vi "HardWareLoop.vi"(8 "error in (no error)":errorcluster, 10 "ctrls":T2, 11 "Queue cluster":T1) -> ()   [LabVIEW 2017]
uses:
  controls_main.ctl
  QueueCluster.ctl
  EventQueueCluster.ctl
  EventMessage.ctl
  MeasureQueue.ctl
  MeasureMessage.ctl
  HardwareQueueCluster.ctl
  hardwareMessage.ctl
  GUIQueueCluster.ctl
  GUIMessage.ctl
  SaveQueueCluster.ctl
  SaveMessage.ctl
  <vilib>/LabVIEW Interface for Arduino/Type Defs/Arduino Resource.ctl
  <vilib>/LabVIEW Interface for Arduino/Type Defs/Board Type.ctl
  <vilib>/LabVIEW Interface for Arduino/LabVIEW Interface for Arduino.lvlib
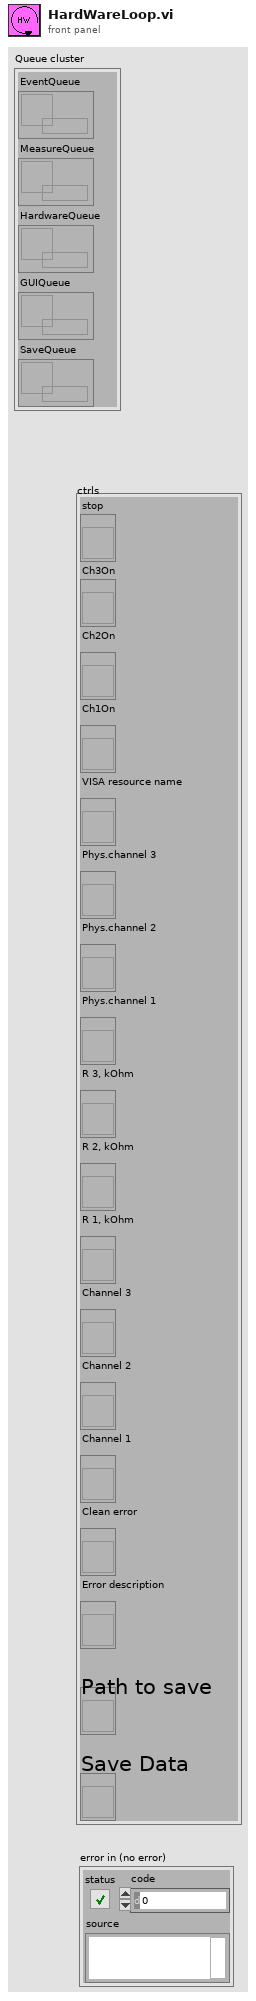
[diagram p1: front panel]
types:
  T1 = typedef "QueueCluster.ctl" = cluster{"EventQueue":refnum<queue>, "MeasureQueue":refnum<queue>, "HardwareQueue":refnum<queue>, "GUIQueue":refnum<queue>, "SaveQueue":refnum<queue>}
  T2 = typedef "controls_main.ctl" = cluster{"stop":refnum<vi>, "Ch3On":refnum<vi>, "Ch2On":refnum<vi>, "Ch1On":refnum<vi>, "VISA resource name":refnum<vi>, "Phys.channel 3":refnum<vi>, "Phys.channel 2":refnum<vi>, "Phys.channel 1":refnum<vi>, "R 3, kOhm":refnum<vi>, "R 2, kOhm":refnum<vi>, "R 1, kOhm":refnum<vi>, "Channel 3":refnum<vi>, "Channel 2":refnum<vi>, "Channel 1":refnum<vi>, "Clean error":refnum<vi>, "Error description":refnum<vi>, "Path to save":refnum<vi>, "Save Data":refnum<vi>}
  T3 = typedef "LabVIEW Interface for Arduino.lvlib/Arduino Resource.ctl" = cluster{"VISA resource":refnum<visa-resource-name>, "Board Type":T4, "Connection Type":enum8{"USB / Serial"}, "Bytes Per Packet (15)":u8}
  T4 = typedef "LabVIEW Interface for Arduino.lvlib/Board Type.ctl" = enum16{"Uno", "Dimuelanove w/Atmega 328", "Mega 2560"}
  T5 = typedef "GUIMessage.ctl" = enum16{"StopSave", "Channel1Value", "Channel2Value", "Channel3Value", "ErrorSource", "CleanError", "StartChannel1", "StartChannel2", "StartChannel3", "StopChannel1", "StopChannel2", "StopChannel3", "Halt"}
  T6 = typedef "GUIQueueCluster.ctl" = cluster{"GUIMessage":T5, "NumericValue":dbl, "String":string}
  T7 = typedef "HardwareQueueCluster.ctl" = cluster{"HardwareMessage":T8, "NumericValue":dbl, "String":string}
  T8 = typedef "hardwareMessage.ctl" = enum16{"Init", "MeasureChannel", "CloseDevice", "Error", "Halt", "SetPhysChannel1", "SetPhysChannel2", "SetPhysChannel3"}
  T9 = typedef "SaveMessage.ctl" = enum16{"StartSaving", "StopSaving", "Ch1Value", "Ch2Value", "Ch3Value", "Error", "WriteFile", "Halt"}
  T10 = typedef "SaveQueueCluster.ctl" = cluster{"Save message":T9, "NumericValue":dbl, "String":string}
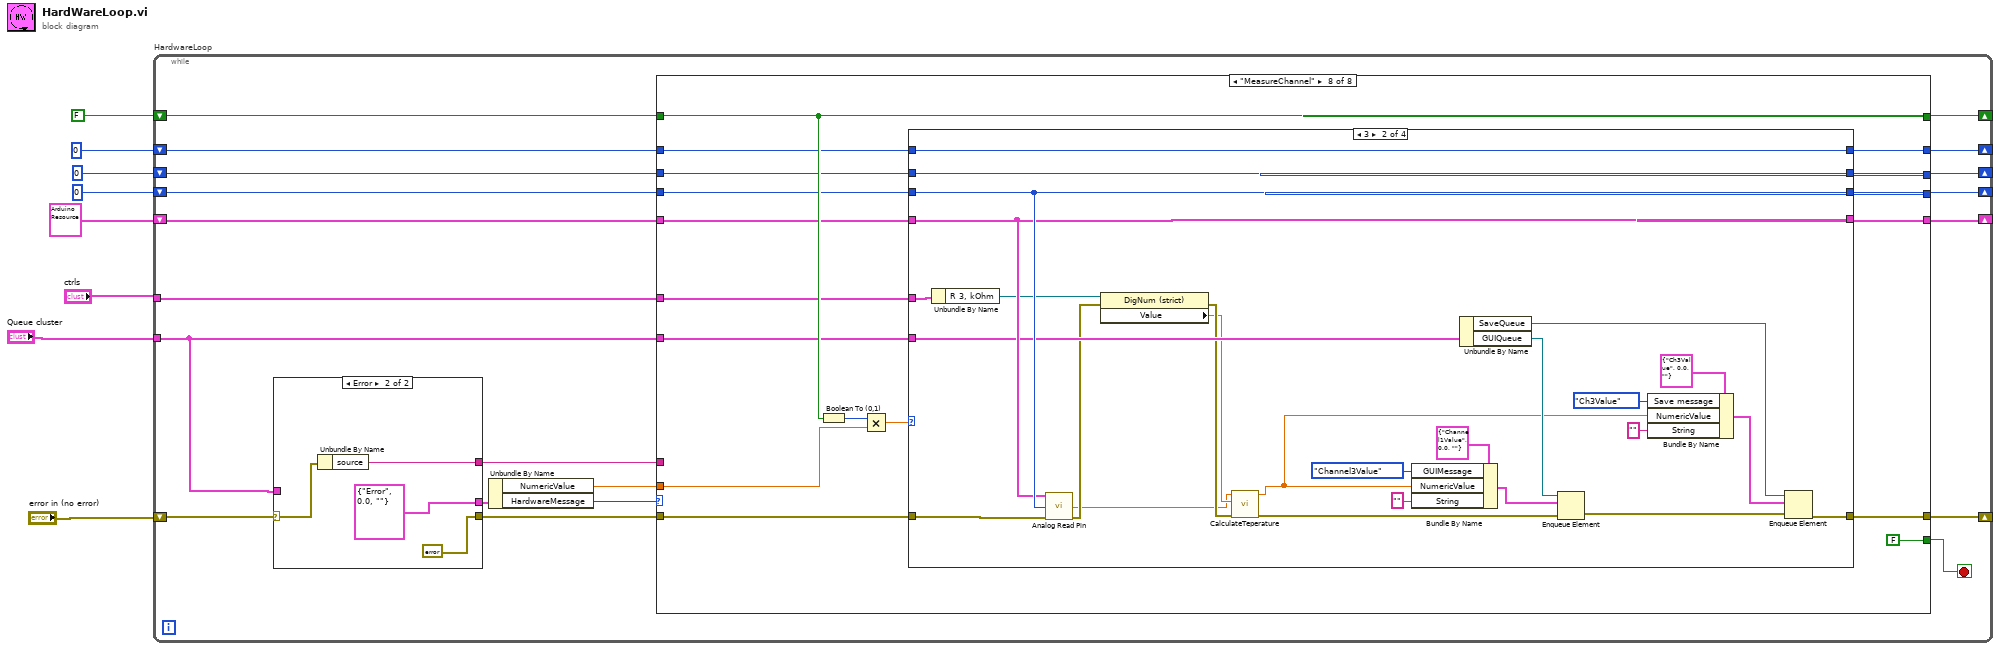
[diagram p0: block diagram]
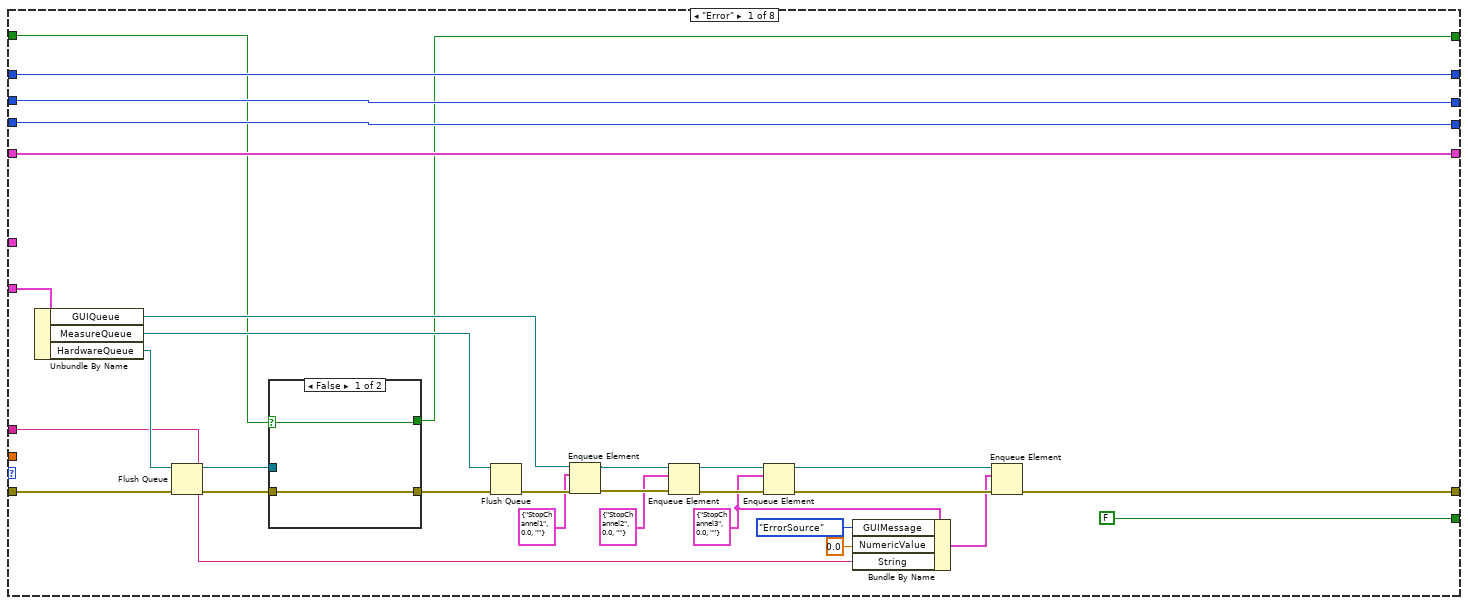
[diagram p2: hidden frame]
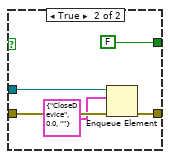
[diagram p3: hidden frame]
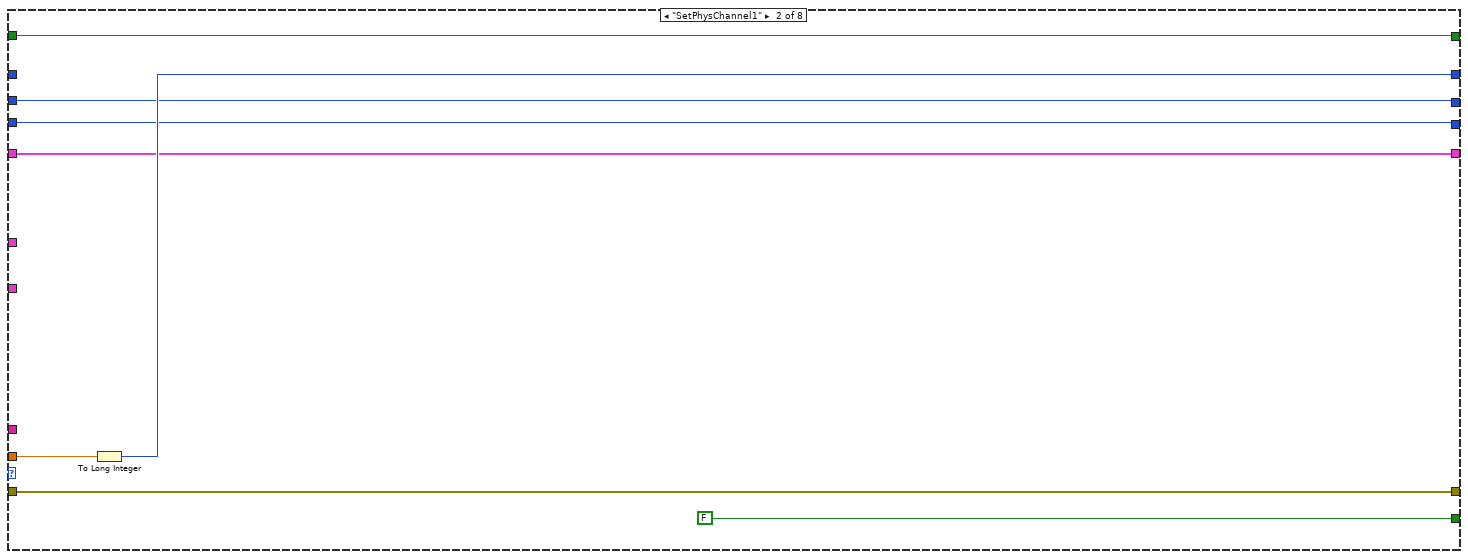
[diagram p4: hidden frame]
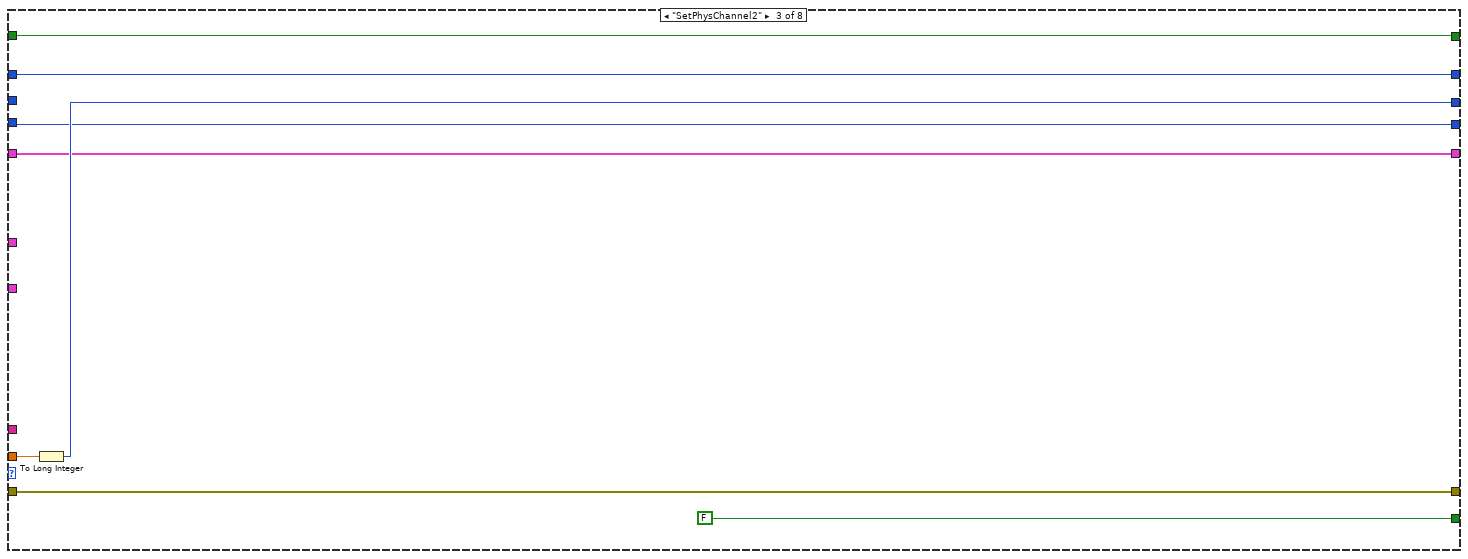
[diagram p5: hidden frame]
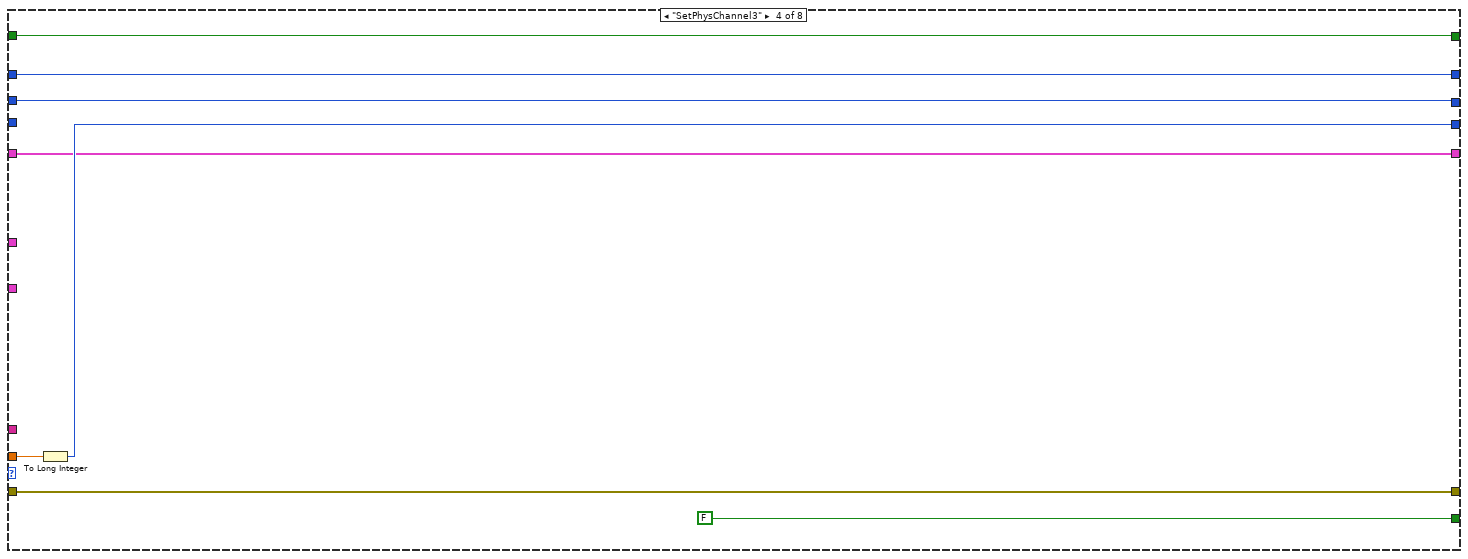
[diagram p6: hidden frame]
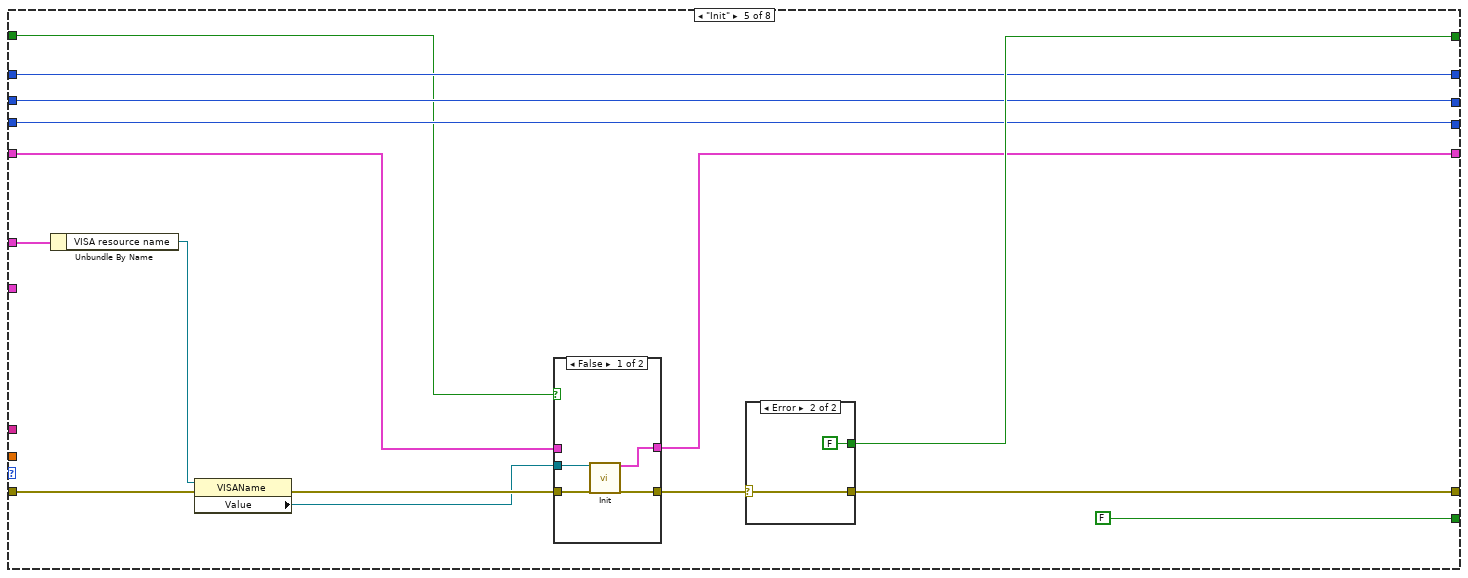
[diagram p7: hidden frame]
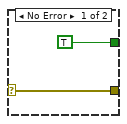
[diagram p9: hidden frame]
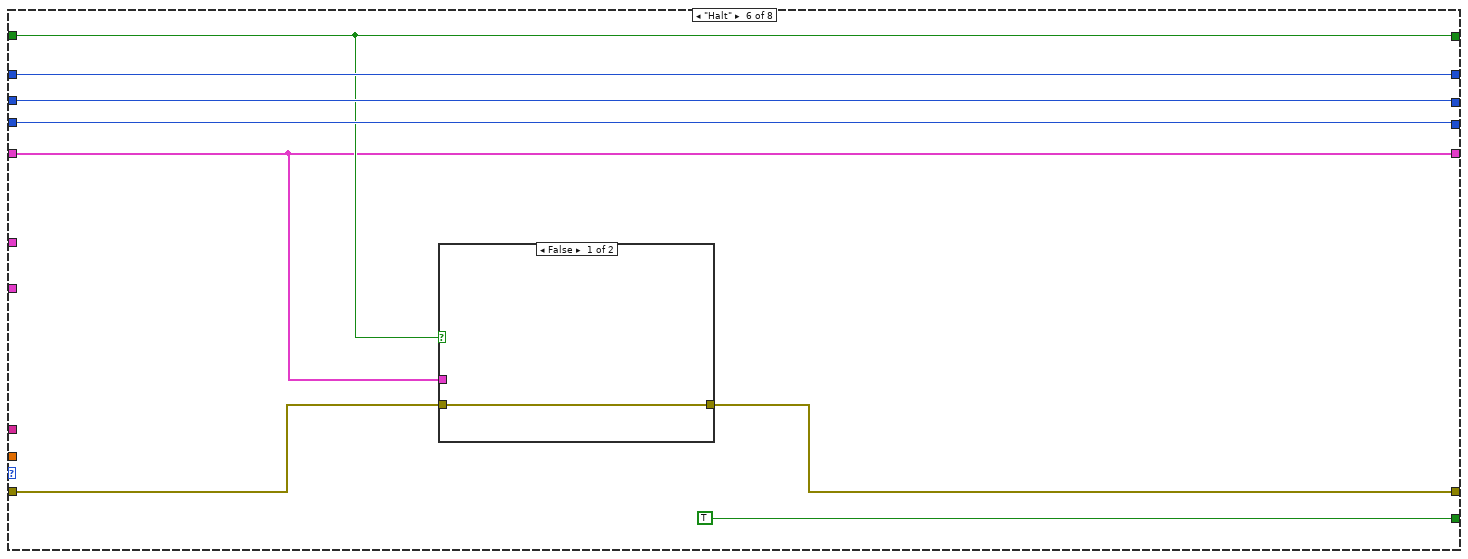
[diagram p10: hidden frame]
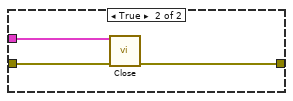
[diagram p11: hidden frame]
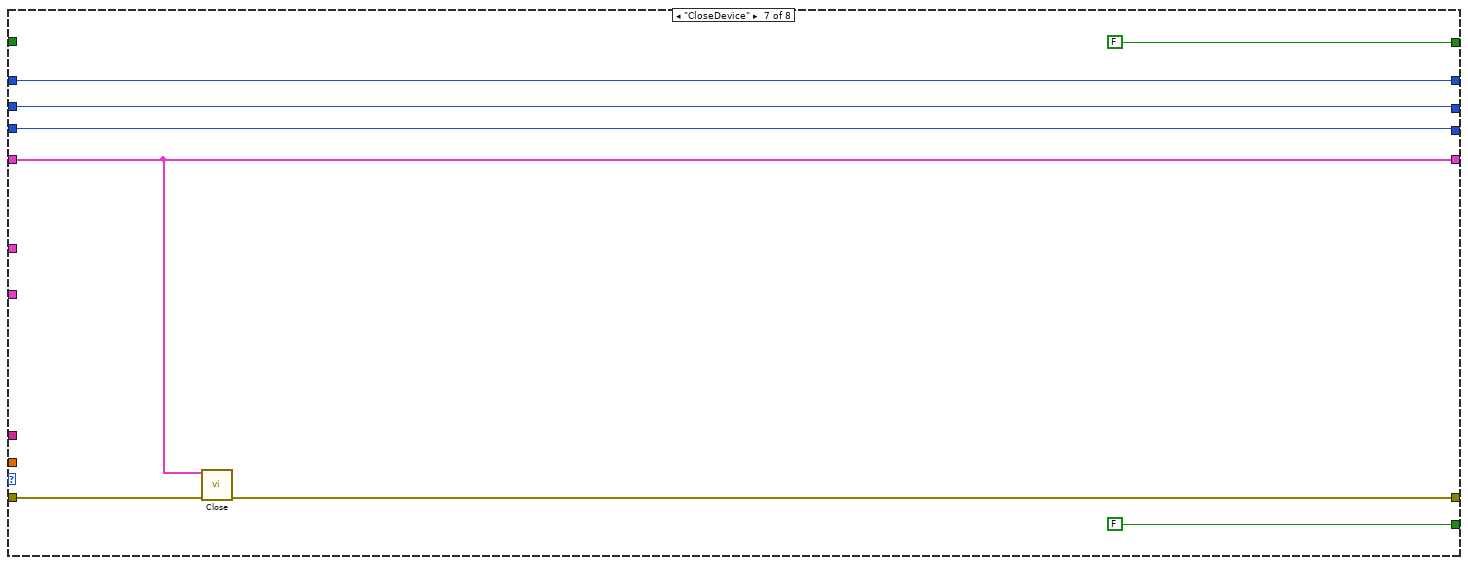
[diagram p12: hidden frame]
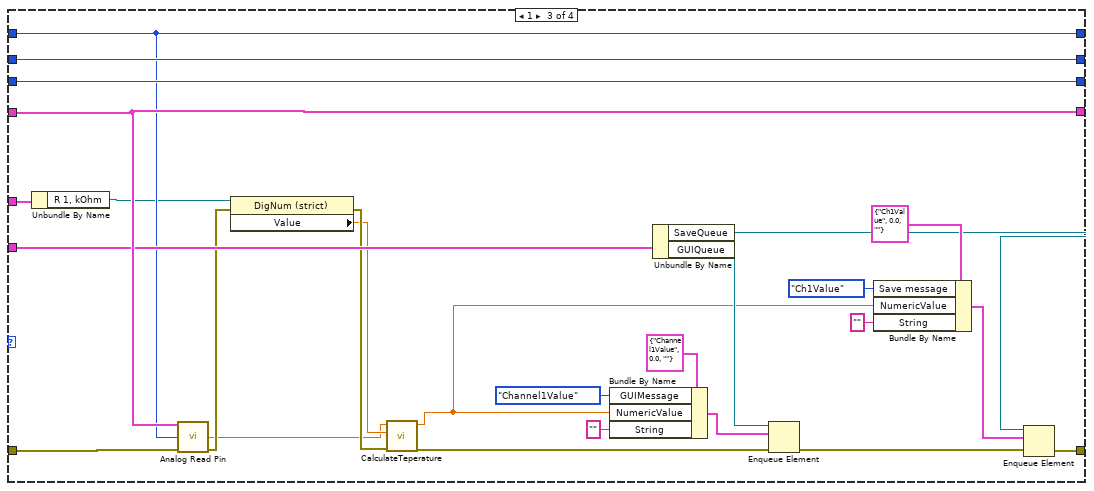
[diagram p14: hidden frame]
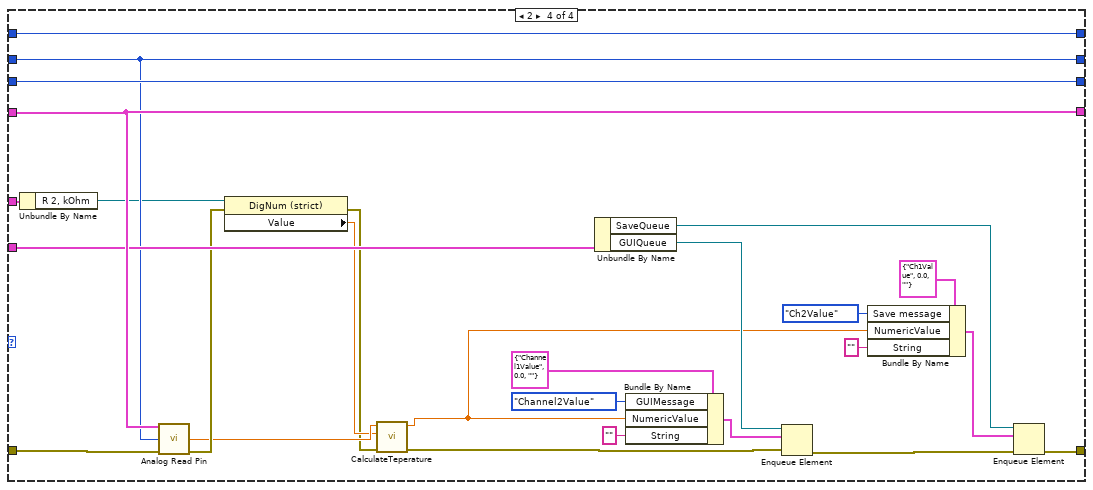
[diagram p15: hidden frame]
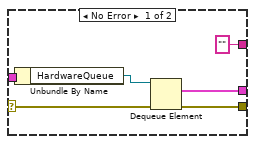
[diagram p16: hidden frame]
diagram:
  n1 = while "HardwareLoop" {
    tunnel: "Queue cluster" -> [w15]
    shift-right: [w14] -> _
    shift-left: "error in (no error)" -> [w28]
    shift-right: [w23] -> _
    shift-left: FALSE -> [w24]
    shift-right: [w19] -> _
    shift-left: 0 -> [w22]
    shift-right: [w18] -> _
    shift-left: 0 -> [w21]
    shift-right: [w17] -> _
    shift-left: 0 -> [w20]
    tunnel: "ctrls" -> [w13]
    shift-right: [w11] -> _
    shift-left: T3 {"VISA resource"="", "Board Type"=enum."Uno", "Connection Type"=enum."USB / Serial", "Bytes Per Packet (15)"=15} ("Arduino Resource") -> [w10]
    stop <- w16 stop-if-true
    n2 = case shown="Error" w28 {
      selector: w28 -> [w238 w243]
      tunnel: w15 -> [w240 _]
      tunnel: [w237 errorcluster {"status"=FALSE, "code"=0, "source"=""} ("error IO")] -> w25
      tunnel: [w236 T7 {"HardwareMessage"=enum."Error", "NumericValue"=0.0, "String"=""} ("HardwareQueueCluster")] -> w27
      tunnel: ["" ("source") w242] -> w9
      frame No Error {
        n3 = Unbundle By Name(w240) -> ("HardwareQueue"=w239:refnum<queue>)
        n4 = Dequeue Element(queue=w239, error in (no error)=w238) -> (element=w236:T7, error out=w237:errorcluster)  [unwired: 1 in, 2 out]
      }
      frame Error {
        n5 = Unbundle By Name(w243) -> ("source"=w242:string)
      }
    }
    n6 = Unbundle By Name(w27) -> ("NumericValue"=w12:dbl, "HardwareMessage"=w26:T8)
    n7 = case shown="\"MeasureChannel\"" w26 {
      tunnel: w25 -> [w53 w69 w76 w84 w96 w116 w134 w151]
      tunnel: w24 -> [w33 w67 w77 w89 w95 w118 _ w147]
      tunnel: [w32 w67 w77 w89 w103 w118 FALSE w147] -> w23
      tunnel: w22 -> [w58 _ w78 w88 w101 w121 w131 w146]
      tunnel: w21 -> [w57 w71 _ w87 w100 w120 w130 w145]
      tunnel: w20 -> [w56 w70 w79 _ w99 w119 w129 w144]
      tunnel: [w58 w72 w78 w88 w101 w121 w131 w141] -> w19
      tunnel: [w57 w71 w80 w87 w100 w120 w130 w140] -> w18
      tunnel: [w56 w70 w79 w85 w99 w119 w129 w139] -> w17
      tunnel: [FALSE FALSE FALSE FALSE FALSE TRUE FALSE FALSE] -> w16
      tunnel: w15 -> [w54 _ _ _ _ _ _ w137]
      tunnel: [w34 w69 w76 w84 w102 w115 w133 w136] -> w14
      tunnel: w13 -> [_ _ _ _ w98 _ _ w135]
      tunnel: w12 -> [_ w73 w81 w86 _ _ _ w149]
      tunnel: [w44 w66 w74 w82 w90 w117 w128 w138] -> w11
      tunnel: w10 -> [w44 w66 w74 w82 w91 w117 w128 w143]
      tunnel: w9 -> [w43 _ _ _ _ _ _ _]
      frame "Error" {
        w37 = T6 {"GUIMessage"=enum."StopChannel3", "NumericValue"=0.0, "String"=""} ("element")
        n8 = Unbundle By Name(w54) -> ("GUIQueue"=w49:refnum<queue>, "MeasureQueue"=w51:refnum<queue>, "HardwareQueue"=w52:refnum<queue>)
        n9 = Flush Queue(queue=w52, error in (no error)=w53) -> (queue out=w31:refnum<queue>, error out=w30:errorcluster)  [unwired: 1 out]
        n10 = case shown="False" w33 {
          selector: w33 -> [w60 _]
          tunnel: [w60 FALSE] -> w32
          tunnel: w31 -> [_ w64]
          tunnel: w30 -> [w59 w63]
          tunnel: [w59 w62] -> w29
          frame False {
          }
          frame True {
            n11 = Enqueue Element(queue=w64, element=T7 {"HardwareMessage"=enum."CloseDevice", "NumericValue"=0.0, "String"=""}, error in (no error)=w63) -> (error out=w62:errorcluster)  [unwired: 1 in, 2 out]
          }
        }
        n12 = Flush Queue(queue=w51, error in (no error)=w29) -> (error out=w50:errorcluster)  [unwired: 2 out]
        n13 = Enqueue Element(queue=w49, element=T6 {"GUIMessage"=enum."StopChannel1", "NumericValue"=0.0, "String"=""}, error in (no error)=w50) -> (queue out=w48:refnum<queue>, error out=w46:errorcluster)  [unwired: 1 in, 1 out]
        n14 = Enqueue Element(queue=w48, element=T6 {"GUIMessage"=enum."StopChannel2", "NumericValue"=0.0, "String"=""}, error in (no error)=w46) -> (queue out=w47:refnum<queue>, error out=w45:errorcluster)  [unwired: 1 in, 1 out]
        n15 = Enqueue Element(queue=w47, element=w37, error in (no error)=w45) -> (queue out=w42:refnum<queue>, error out=w41:errorcluster)  [unwired: 1 in, 1 out]
        n16 = Bundle By Name(cluster=w37, "GUIMessage"=GUIMessage."ErrorSource", "NumericValue"=0.0, "String"=w43) -> (w35:T6)
        n17 = Enqueue Element(queue=w42, element=w35, error in (no error)=w41) -> (error out=w34:errorcluster)  [unwired: 1 in, 2 out]
      }
      frame "SetPhysChannel1" {
        n18 = To Long Integer(number=w73) -> (32bit integer=w72:i32)
      }
      frame "SetPhysChannel2" {
        n19 = To Long Integer(number=w81) -> (32bit integer=w80:i32)
      }
      frame "SetPhysChannel3" {
        n20 = To Long Integer(number=w86) -> (32bit integer=w85:i32)
      }
      frame "Init" {
        n21 = Unbundle By Name(w98) -> ("VISA resource name"=w97:refnum<vi>)
        n22 = property class="VISAName"(reference=w97, error in=w96) -> (error out=w94:errorcluster, "Value"=w92:refnum<visa-resource-name>)  [unwired: 1 out]
        n23 = case shown="False" w95 {
          tunnel: w94 -> [w108 w110]
          tunnel: [w107 w110] -> w93
          tunnel: w92 -> [w106 _]
          tunnel: [w105 w109] -> w90
          tunnel: w91 -> [_ w109]
          frame False {
            n24 = call <vilib>:"Init.vi"("VISA resource"=w106, "error in"=w108) -> ("Arduino Resource"=w105:T3, "error out"=w107:errorcluster)  [unwired: 16 in]
          }
          frame True {
          }
        }
        n25 = case shown="Error" w93 {
          selector: w93 -> [w111 w113]
          tunnel: [TRUE FALSE] -> w103
          tunnel: [w111 w113] -> w102
          frame No Error {
          }
          frame Error {
          }
        }
      }
      frame "Halt" {
        n26 = case shown="False" w118 {
          tunnel: w117 -> [_ w126]
          tunnel: w116 -> [w123 w125]
          tunnel: [w123 w124] -> w115
          frame False {
          }
          frame True {
            n27 = call <vilib>:"Close.vi"("Arduino Resource"=w126, "error in"=w125) -> ("error out"=w124:errorcluster)  [unwired: 13 in]
          }
        }
      }
      frame "CloseDevice" {
        n28 = call <vilib>:"Close.vi"("Arduino Resource"=w128, "error in"=w134) -> ("error out"=w133:errorcluster)  [unwired: 13 in]
      }
      frame "MeasureChannel" {
        n29 = Boolean To (0,1)(Boolean=w147) -> (0, 1=w150:i16)
        n30 = Multiply(x=w150, y=w149) -> (x*y=w148:dbl)
        n31 = case shown="3" w148 {
          tunnel: w151 -> [w152 w182 w208 w234]
          tunnel: w146 -> [w156 w181 w198 w233]
          tunnel: w145 -> [w155 w180 w207 w224]
          tunnel: w144 -> [w154 w179 w206 w232]
          tunnel: w143 -> [w153 w178 w205 w231]
          tunnel: [w156 w181 w198 w233] -> w141
          tunnel: [w155 w180 w207 w224] -> w140
          tunnel: [w154 w179 w206 w232] -> w139
          tunnel: [w153 w178 w205 w231] -> w138
          tunnel: w137 -> [_ w176 w203 w229]
          tunnel: [w152 w170 w192 w217] -> w136
          tunnel: w135 -> [_ w164 w190 w216]
          frame 0, Default {
          }
          frame 3 {
            n32 = Unbundle By Name(w164) -> ("R 3, kOhm"=w163:refnum<vi>)
            n33 = call <vilib>:"Analog Read Pin.vi"("Arduino Resource"=w178, "Analog Input Pin (0)"=w179, "error in"=w182) -> ("Voltage"=w159:dbl, "error out"=w162:errorcluster)  [unwired: 10 in, 1 out]
            n34 = property class="DigNum (strict)"(reference=w163, error in=w162) -> (error out=w161:errorcluster, "Value"=w160:dbl)  [unwired: 1 out]
            n35 = call "CalculateTeperature.vi"("error in (no error)"=w161, "Resistor"=w160, "ChannelVoltage"=w159) -> ("error out"=w158:errorcluster, "Temperature"=w157:dbl)  [unwired: 7 in]
            n36 = Bundle By Name(cluster=T6 {"GUIMessage"=enum."Channel1Value", "NumericValue"=0.0, "String"=""} ("element"), "GUIMessage"=GUIMessage."Channel3Value", "NumericValue"=w157, "String"="") -> (w172:T6)
            n37 = Unbundle By Name(w176) -> ("SaveQueue"=w169:refnum<queue>, "GUIQueue"=w177:refnum<queue>)
            n38 = Enqueue Element(queue=w177, element=w172, error in (no error)=w158) -> (error out=w171:errorcluster)  [unwired: 1 in, 2 out]
            n39 = Bundle By Name(cluster=T10 {"Save message"=enum."Ch3Value", "NumericValue"=0.0, "String"=""} ("element"), "Save message"=SaveMessage."Ch3Value", "NumericValue"=w157, "String"="") -> (w165:T10)
            n40 = Enqueue Element(queue=w169, element=w165, error in (no error)=w171) -> (error out=w170:errorcluster)  [unwired: 1 in, 2 out]
          }
          frame 1 {
            n41 = Unbundle By Name(w190) -> ("R 1, kOhm"=w189:refnum<vi>)
            n42 = call <vilib>:"Analog Read Pin.vi"("Arduino Resource"=w205, "Analog Input Pin (0)"=w198, "error in"=w208) -> ("Voltage"=w184:dbl, "error out"=w188:errorcluster)  [unwired: 10 in, 1 out]
            n43 = property class="DigNum (strict)"(reference=w189, error in=w188) -> (error out=w187:errorcluster, "Value"=w186:dbl)  [unwired: 1 out]
            n44 = call "CalculateTeperature.vi"("error in (no error)"=w187, "Resistor"=w186, "ChannelVoltage"=w184) -> ("error out"=w185:errorcluster, "Temperature"=w183:dbl)  [unwired: 7 in]
            n45 = Bundle By Name(cluster=T6 {"GUIMessage"=enum."Channel1Value", "NumericValue"=0.0, "String"=""} ("element"), "GUIMessage"=GUIMessage."Channel1Value", "NumericValue"=w183, "String"="") -> (w199:T6)
            n46 = Unbundle By Name(w203) -> ("SaveQueue"=w191:refnum<queue>, "GUIQueue"=w204:refnum<queue>)
            n47 = Enqueue Element(queue=w204, element=w199, error in (no error)=w185) -> (error out=w193:errorcluster)  [unwired: 1 in, 2 out]
            n48 = Bundle By Name(cluster=T10 {"Save message"=enum."Ch1Value", "NumericValue"=0.0, "String"=""} ("element"), "Save message"=SaveMessage."Ch1Value", "NumericValue"=w183, "String"="") -> (w194:T10)
            n49 = Enqueue Element(queue=w191, element=w194, error in (no error)=w193) -> (error out=w192:errorcluster)  [unwired: 1 in, 2 out]
          }
          frame 2 {
            n50 = Unbundle By Name(w216) -> ("R 2, kOhm"=w215:refnum<vi>)
            n51 = call <vilib>:"Analog Read Pin.vi"("Arduino Resource"=w231, "Analog Input Pin (0)"=w224, "error in"=w234) -> ("Voltage"=w213:dbl, "error out"=w214:errorcluster)  [unwired: 10 in, 1 out]
            n52 = property class="DigNum (strict)"(reference=w215, error in=w214) -> (error out=w211:errorcluster, "Value"=w212:dbl)  [unwired: 1 out]
            n53 = call "CalculateTeperature.vi"("error in (no error)"=w211, "Resistor"=w212, "ChannelVoltage"=w213) -> ("error out"=w210:errorcluster, "Temperature"=w209:dbl)  [unwired: 7 in]
            n54 = Unbundle By Name(w229) -> ("SaveQueue"=w218:refnum<queue>, "GUIQueue"=w230:refnum<queue>)
            n55 = Bundle By Name(cluster=T6 {"GUIMessage"=enum."Channel1Value", "NumericValue"=0.0, "String"=""} ("element"), "GUIMessage"=GUIMessage."Channel2Value", "NumericValue"=w209, "String"="") -> (w225:T6)
            n56 = Enqueue Element(queue=w230, element=w225, error in (no error)=w210) -> (error out=w219:errorcluster)  [unwired: 1 in, 2 out]
            n57 = Bundle By Name(cluster=T10 {"Save message"=enum."Ch1Value", "NumericValue"=0.0, "String"=""} ("element"), "Save message"=SaveMessage."Ch2Value", "NumericValue"=w209, "String"="") -> (w220:T10)
            n58 = Enqueue Element(queue=w218, element=w220, error in (no error)=w219) -> (error out=w217:errorcluster)  [unwired: 1 in, 2 out]
          }
        }
      }
    }
  }
